vi "PopulatePad.vi"(7 "Pad":string, 8 "error in (no error)":errorcluster, 9 "PadArea":T1, 10 "Set Pad?":bool, 11 "EpiWrapper in":refnum<class "EpiWrapper.lvclass">) -> (0 "error out":errorcluster, 3 "EpiWrapper out":refnum<class "EpiWrapper.lvclass">)   [LabVIEW 2012, in "EpiWrapper.lvclass"]
uses:
  EpiWrapper.lvclass
  Controls/PadArea.ctl
  EpiWrapper.lvclass/EpiWrapper.ctl
  PadLookupVar.vi
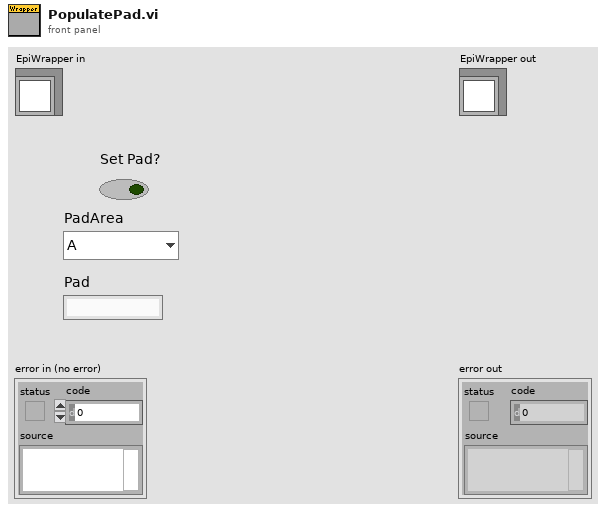
[diagram p1: front panel]
types:
  T1 = typedef "PadArea.ctl" = enum16{"A", "B", "C", "D", "L", "R", "T", "G"}
  T2 = typedef "PadLookup.ctl" = cluster{"A":T3, "B":T3, "C":T3, "D":T3, "L":T3, "R":T3, "T":T3, "G":T3}
  T3 = typedef "PadLookupItem.ctl" = cluster{"PadArea":T1, string[]}
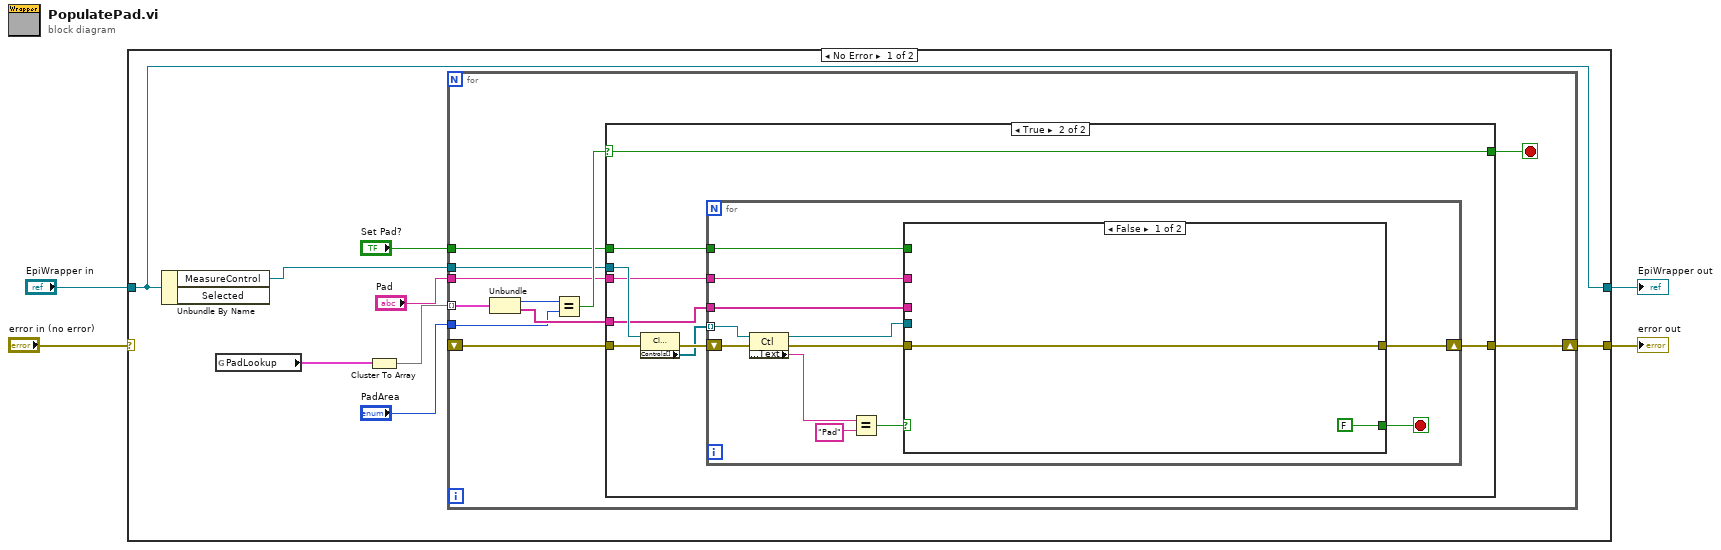
[diagram p0: block diagram]
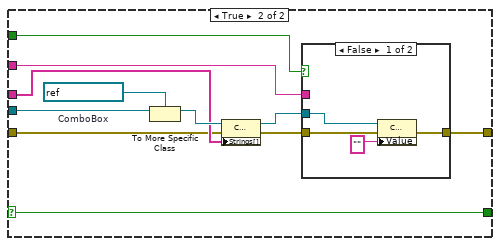
[diagram p3: hidden frame]
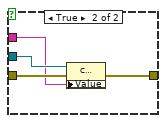
[diagram p4: hidden frame]
diagram:
  n1 = case shown="No Error" "error in (no error)" {
    selector: "error in (no error)" -> [_ w69]
    tunnel: [w7 w69] -> w3
    tunnel: [w6 w68] -> w1
    tunnel: "EpiWrapper in" -> [w6 w68]
    frame No Error {
      n2 = Unbundle By Name(w6) -> ("MeasureControl"=w8:refnum<vi>)  [unwired: 1 out]
      n3 = global read "PadLookupVar.vi" "PadLookup"() -> (w5:T2)
      n4 = Cluster To Array(cluster=w5) -> (array=w12:T3[])
      n5 = for {
        tunnel: w12 -> [w23] mode=indexing
        tunnel: "PadArea" -> [w18]
        tunnel: w8 -> [w17]
        tunnel: "Set Pad?" -> [w16]
        tunnel: "Pad" -> [w15]
        shift-right: [w14] -> w7
        shift-left: _ -> [w13]
        stop <- w20 stop-if-true
        n6 = Unbundle(w23) -> ("PadArea"=w22:T1, w19:string[])
        n7 = Equal?(x=w22, y=w18) -> (x = y?=w21:bool)
        n8 = case shown="True" w21 {
          selector: w21 -> [w25 w34]
          tunnel: [w25 w34] -> w20
          tunnel: w19 -> [_ w30]
          tunnel: w17 -> [_ w31]
          tunnel: w16 -> [_ w29]
          tunnel: w15 -> [_ w28]
          tunnel: [w24 w27] -> w14
          tunnel: w13 -> [w24 w26]
          frame False {
          }
          frame True {
            n9 = property class="Clust (strict)"(reference=w31, error in=w26) -> (error out=w33:errorcluster, "Controls[]"=w32:refnum<vi>[])  [unwired: 1 out]
            n10 = for {
              tunnel: w32 -> [w46] mode=indexing
              tunnel: w30 -> [w41]
              tunnel: w29 -> [w37]
              tunnel: w28 -> [w36]
              shift-right: [w35] -> w27
              shift-left: w33 -> [w39]
              stop <- w38 stop-if-true
              n11 = property class="Ctl"(reference=w46, error in=w39) -> (reference out=w42:refnum<vi>, error out=w40:errorcluster, "Label.Text"=w45:string)
              n12 = Equal?(x=w45, y="Pad") -> (x = y?=w43:bool)
              n13 = case shown="False" w43 {
                selector: w43 -> [_ w54]
                tunnel: w42 -> [_ w59]
                tunnel: w41 -> [_ w56]
                tunnel: w40 -> [w47 w55]
                tunnel: [FALSE w54] -> w38
                tunnel: w37 -> [_ w53]
                tunnel: w36 -> [_ w50]
                tunnel: [w47 w49] -> w35
                frame False {
                }
                frame True {
                  w58 = refnum<vi> refnum  # ComboBox
                  n14 = To More Specific Class(target class=w58, reference=w59) -> (specific class reference=w57:refnum<vi>)  [unwired: 1 in, 1 out]
                  n15 = property class="CmbBox"(reference=w57, error in=w55, "Strings[]"=w56) -> (reference out=w52:refnum<vi>, error out=w51:errorcluster)
                  n16 = case shown="False" w53 {
                    tunnel: w52 -> [w62 w67]
                    tunnel: w51 -> [w61 w66]
                    tunnel: w50 -> [_ w65]
                    tunnel: [w60 w64] -> w49
                    frame False {
                      n17 = property class="CmbBox"(reference=w62, error in=w61, "Value"="") -> (error out=w60:errorcluster)  [unwired: 1 out]
                    }
                    frame True {
                      n18 = property class="CmbBox"(reference=w67, error in=w66, "Value"=w65) -> (error out=w64:errorcluster)  [unwired: 1 out]
                    }
                  }
                }
              }
            }
          }
        }
      }
    }
    frame Error {
    }
  }
  "error out" <- w3
  "EpiWrapper out" <- w1
